vi "TrajectoryBegin.vi"(8 "error in (no error)":errorcluster) -> (0 "error out":errorcluster)   [LabVIEW 2023]
uses:
  TrajectoryGlobals.vi
  <vilib>/Rock Robotics/WPI/ThirdParty/JAS_Junk/TrajLib/Trajectory_Library.lvlib
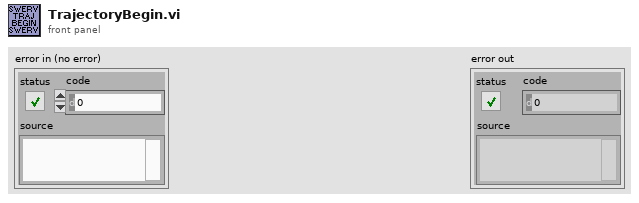
[diagram p1: front panel]
types:
  T1 = typedef "Trajectory_Library.lvlib/TRAJECTORY.ctl" = cluster{"TotalTImeSecs":dbl, "States":T2[]}
  T2 = typedef "Trajectory_Library.lvlib/TRAJ_STATE.ctl" = cluster{"TimeSeconds":dbl, "Velocity":dbl, "Acceleration":dbl, "POSE":T3, "Curvature":dbl}
  T3 = typedef "Trajectory_Library.lvlib/POSE2D.ctl" = cluster{"TRANSLATION":T4, "ROTATION":T5}
  T4 = typedef "Trajectory_Library.lvlib/TRANSLATION2D.ctl" = cluster{"X":dbl, "Y":dbl}
  T5 = typedef "Trajectory_Library.lvlib/ROTATION2D.ctl" = cluster{"VALUE":dbl, "COS":dbl, "SIN":dbl}
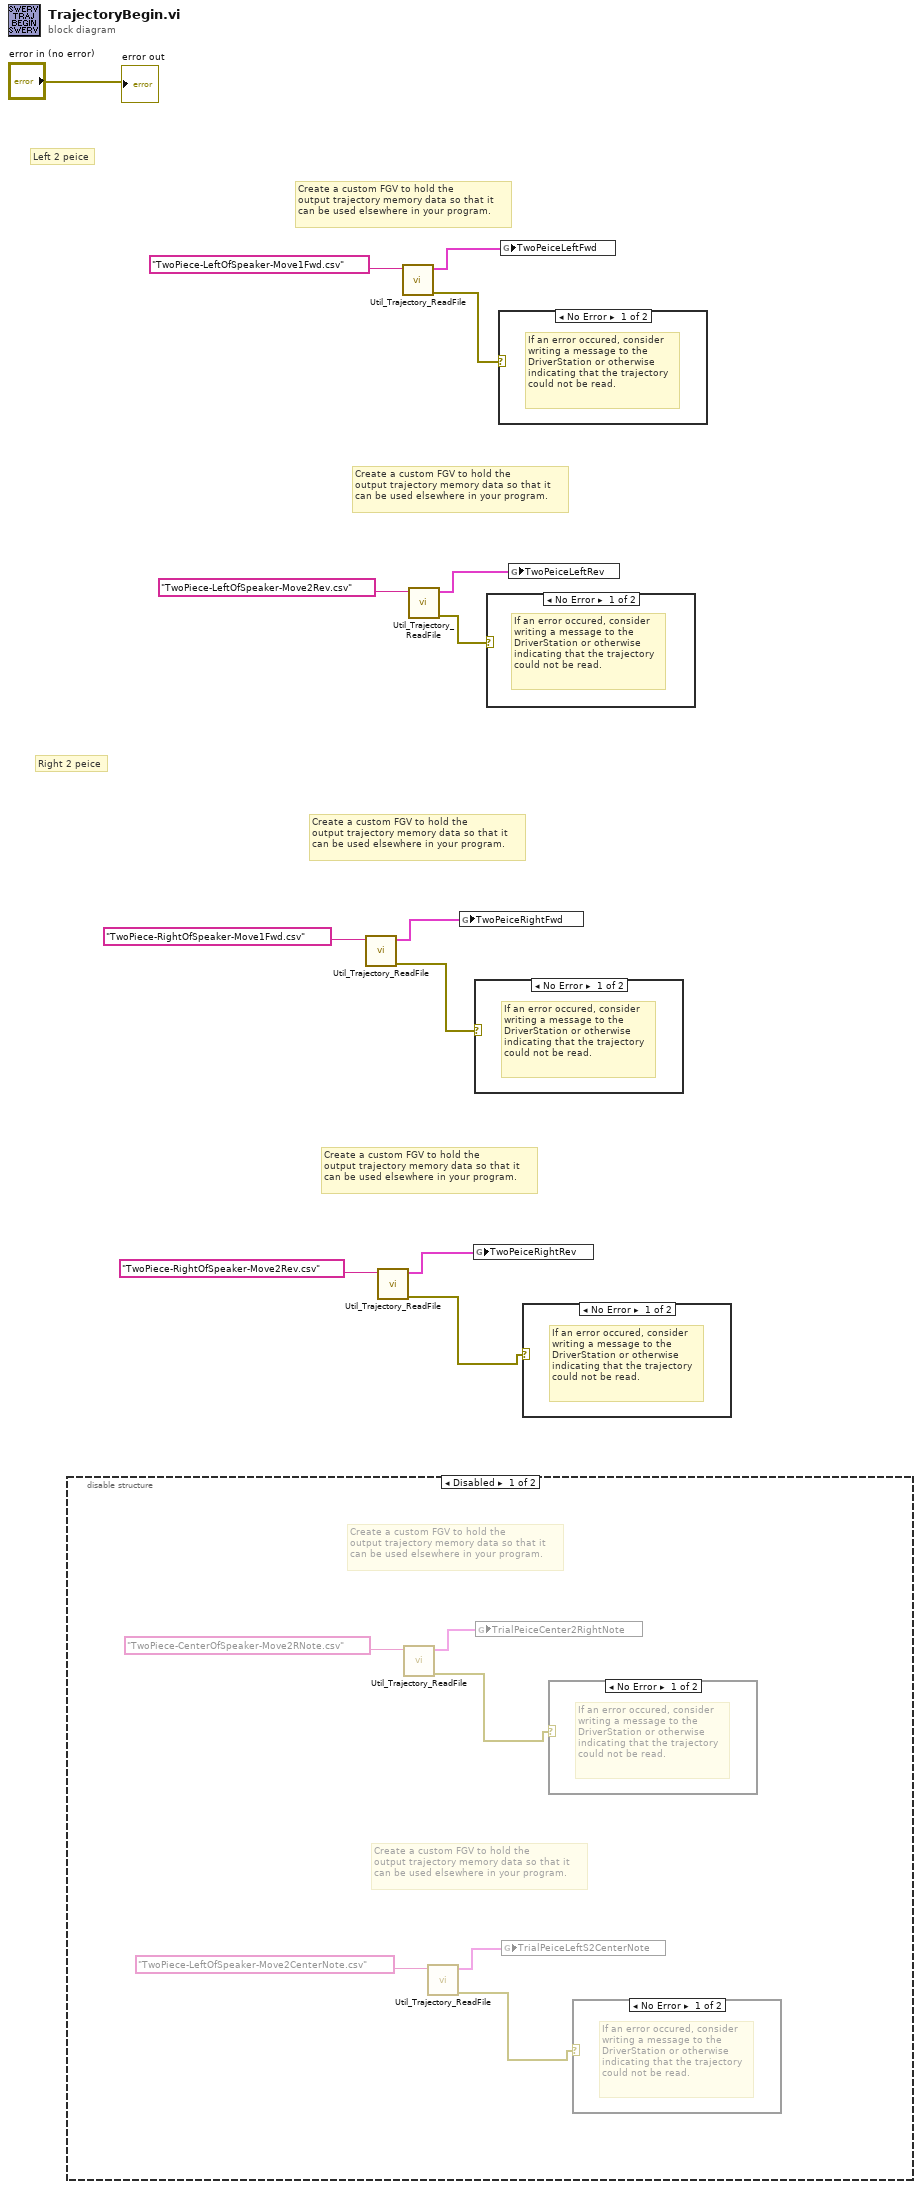
[diagram p0: block diagram]
diagram:
  # "Right 2 peice"
  # "Left 2 peice"
  # "Create a custom FGV to hold the \noutput trajectory memory data so that it\ncan be used elsewhere in your program."
  # "Create a custom FGV to hold the \noutput trajectory memory data so that it\ncan be used elsewhere in your program."
  # "Create a custom FGV to hold the \noutput trajectory memory data so that it\ncan be used elsewhere in your program."
  # "Create a custom FGV to hold the \noutput trajectory memory data so that it\ncan be used elsewhere in your program."
  n1 = disable-structure shown="Disabled" {
    frame Disabled {
      # "Create a custom FGV to hold the \noutput trajectory memory data so that it\ncan be used elsewhere in your program."
      # "Create a custom FGV to hold the \noutput trajectory memory data so that it\ncan be used elsewhere in your program."
      n2 = call <vilib>:"Util_Trajectory_ReadFile.vi"("FileName"="TwoPiece-CenterOfSpeaker-Move2RNote.csv") -> ("error out"=w17:errorcluster, "outTRAJECTORY"=w18:T1)  [unwired: 8 in, 1 out]
      n3 = call <vilib>:"Util_Trajectory_ReadFile.vi"("FileName"="TwoPiece-LeftOfSpeaker-Move2CenterNote.csv") -> ("error out"=w14:errorcluster, "outTRAJECTORY"=w15:T1)  [unwired: 8 in, 1 out]
      n4 = global write "TrajectoryGlobals.vi" "TrialPeiceCenter2RightNote"(w18) -> ()
      n5 = global write "TrajectoryGlobals.vi" "TrialPeiceLeftS2CenterNote"(w15) -> ()
      n6 = case shown="No Error" w17 {
        frame No Error {
          # "If an error occured, consider\nwriting a message to the\nDriverStation or otherwise\nindicating that the trajectory\ncould not be read."
        }
        frame Error {
        }
      }
      n7 = case shown="No Error" w14 {
        frame No Error {
          # "If an error occured, consider\nwriting a message to the\nDriverStation or otherwise\nindicating that the trajectory\ncould not be read."
        }
        frame Error {
        }
      }
    }
    frame Enabled {
    }
  }
  n8 = call <vilib>:"Util_Trajectory_ReadFile.vi"("FileName"="TwoPiece-RightOfSpeaker-Move1Fwd.csv") -> ("error out"=w4:errorcluster, "outTRAJECTORY"=w5:T1)  [unwired: 8 in, 1 out]
  n9 = call <vilib>:"Util_Trajectory_ReadFile.vi"("FileName"="TwoPiece-RightOfSpeaker-Move2Rev.csv") -> ("error out"=w1:errorcluster, "outTRAJECTORY"=w2:T1)  [unwired: 8 in, 1 out]
  n10 = call <vilib>:"Util_Trajectory_ReadFile.vi"("FileName"="TwoPiece-LeftOfSpeaker-Move1Fwd.csv") -> ("error out"=w12:errorcluster, "outTRAJECTORY"=w10:T1)  [unwired: 8 in, 1 out]
  n11 = call <vilib>:"Util_Trajectory_ReadFile.vi"("FileName"="TwoPiece-LeftOfSpeaker-Move2Rev.csv") -> ("error out"=w7:errorcluster, "outTRAJECTORY"=w8:T1)  [unwired: 8 in, 1 out]
  n12 = global write "TrajectoryGlobals.vi" "TwoPeiceRightFwd"(w5) -> ()
  n13 = global write "TrajectoryGlobals.vi" "TwoPeiceRightRev"(w2) -> ()
  n14 = case shown="No Error" w4 {
    frame No Error {
      # "If an error occured, consider\nwriting a message to the\nDriverStation or otherwise\nindicating that the trajectory\ncould not be read."
    }
    frame Error {
    }
  }
  n15 = case shown="No Error" w7 {
    frame No Error {
      # "If an error occured, consider\nwriting a message to the\nDriverStation or otherwise\nindicating that the trajectory\ncould not be read."
    }
    frame Error {
    }
  }
  n16 = case shown="No Error" w12 {
    frame No Error {
      # "If an error occured, consider\nwriting a message to the\nDriverStation or otherwise\nindicating that the trajectory\ncould not be read."
    }
    frame Error {
    }
  }
  n17 = global write "TrajectoryGlobals.vi" "TwoPeiceLeftFwd"(w10) -> ()
  n18 = global write "TrajectoryGlobals.vi" "TwoPeiceLeftRev"(w8) -> ()
  n19 = case shown="No Error" w1 {
    frame No Error {
      # "If an error occured, consider\nwriting a message to the\nDriverStation or otherwise\nindicating that the trajectory\ncould not be read."
    }
    frame Error {
    }
  }
  "error out" <- "error in (no error)"
